vi "ScaleGetErr.vi"(2 "error code":i32, 3 "error in":errorcluster) -> (1 "error out":errorcluster)   [LabVIEW 2017]
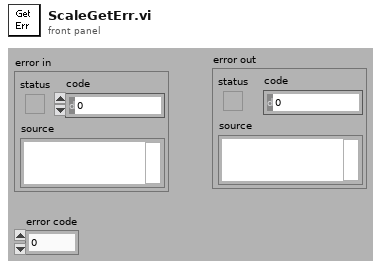
[diagram p1: front panel]
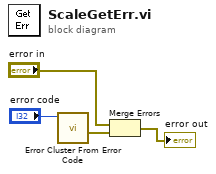
[diagram p0: block diagram]
diagram:
  n1 = call <vilib>:"Error Cluster From Error Code.vi"("error code (0)"="error code") -> ("error out"=w4:errorcluster)  [unwired: 2 in, 6 out]
  n2 = Merge Errors("error in", w4) -> (→"error out":errorcluster)
